vi "禹山pH_获取温度和测量值.vi"(8 "error in (no error)":errorcluster caption="错误输入（无错误）", 11 "MB session in":refnum<class "MB_Master.lvclass">) -> (0 "error out":errorcluster caption="错误输出", 2 "输出值":cluster{"温度测量值":sgl, "ORP":sgl, "pH":sgl}, 3 "MB session out":refnum<class "MB_Master.lvclass">)   [LabVIEW 2016, in "斯坦道多参数.lvlib"]
uses:
  <vilib>/Plasmionique/MB Master/MB_Master/MB_Master.lvclass
  <vilib>/Plasmionique/MB Master/MB Master.lvlib
  <vilib>/ptbypt/NI_PtbyPt.lvlib
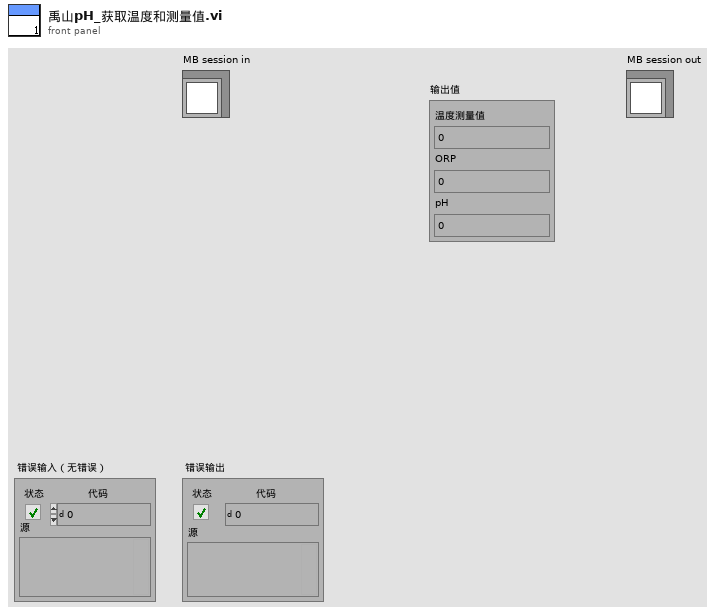
[diagram p1: front panel]
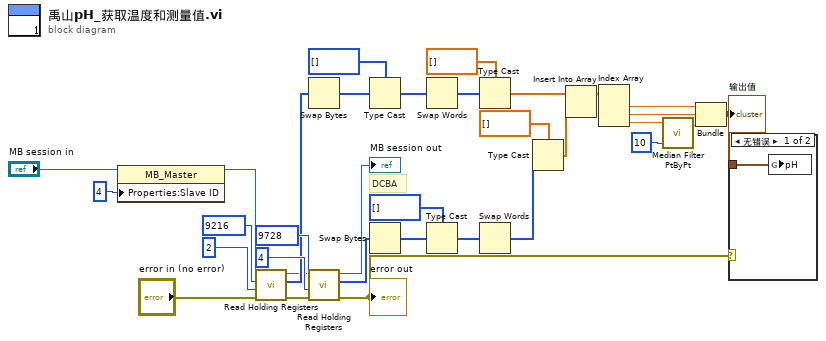
[diagram p0: block diagram]
diagram:
  # "DCBA"
  n1 = property class="MB_Master"(reference="MB session in", "Properties:Slave ID"=u16 4 ("y")) -> (reference out=w10:refnum<class "MB_Master.lvclass">)  [unwired: 1 in, 1 out]
  n2 = call <vilib>:"Read Holding Registers.vi"("error in (no error)"="error in (no error)", "quantity"=u16 2, "starting address"=u16 9216, "MB session in"=w10) -> ("error out"=w11:errorcluster, "Registers"=w14:u16[], "MB session out"=w9:refnum<class "MB_Master.lvclass">)  [unwired: 5 in]
  n3 = Swap Bytes(anything=w14) -> (byte swapped=w19:u16[])
  n4 = call <vilib>:"Read Holding Registers.vi"("error in (no error)"=w11, "quantity"=u16 4, "starting address"=u16 9728, "MB session in"=w9) -> ("error out"=w13:errorcluster, "Registers"=w26:u16[], "MB session out"=→"MB session out":refnum<class "MB_Master.lvclass">)  [unwired: 5 in]
  "error out" <- w13
  n5 = Type Cast(type=u32[] [] ("数组 2"), x=w19) -> (*(type *) &x=w17:u32[])
  n6 = Swap Bytes(anything=w26) -> (byte swapped=w25:u16[])
  n7 = Swap Words(1:w17) -> (0:w15:u32[])
  n8 = Type Cast(type=u32[] [] ("数组 2"), x=w25) -> (*(type *) &x=w29:u32[])
  n9 = Type Cast(type=sgl[] [] ("数组 2"), x=w15) -> (*(type *) &x=w8:sgl[])
  n10 = Swap Words(1:w29) -> (0:w31:u32[])
  n11 = Type Cast(type=sgl[] [] ("数组 2"), x=w31) -> (*(type *) &x=w6:sgl[])
  n12 = Insert Into Array(array=w8, new element=w6) -> (w7:sgl[])  [unwired: 1 in]
  n13 = Index Array(array=w7) -> (element #1=w24:sgl, element #2=w23:sgl, element #3=w2:sgl)  [unwired: 3 in]
  n14 = call <vilib>:"Median Filter PtByPt.vi"("rank"=10, "x"=w2) -> ("Filtered x"=w1:dbl)  [unwired: 2 in, 1 out]
  n15 = Bundle("数值"=w24, "数值"=w23, "Filtered x"=w1) -> (w22:cluster{"数值":sgl, "数值":sgl, "Filtered x":dbl})  [unwired: 1 in]
  "输出值" <- w22
  n16 = case shown="无错误" w13 {
    tunnel: w22 -> [w34 _]
    frame No Error {
      n17 = global write "禹山过程全局变量.vi" "pH"(w34) -> ()
    }
    frame Error {
    }
  }
